vi "Circular Buffer Address.vi"(5 "Reset?":bool, 7 "Starting Address":u32, 11 "Records to Acquire":u32) -> (3 "Address":u32)   [LabVIEW 2012]
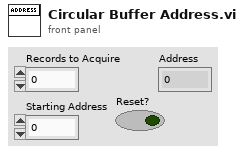
[diagram p1: front panel]
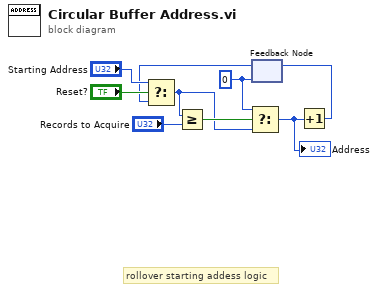
[diagram p0: block diagram]
diagram:
  w9 = u32 0
  # "rollover starting addess logic"
  n1 = feedback #1(w9) -> (w2:u32)
  n2 = Select(t="Starting Address", s="Reset?", f=w2) -> (s? t:f=w1:u32)
  n3 = Greater Or Equal?(x=w1, y="Records to Acquire") -> (x >= y?=w8:bool)
  n4 = Select(t=w9, s=w8, f=w1) -> (s? t:f=w3:u32)
  "Address" <- w3
  n5 = Increment(x=w3) -> (x+1=w6:u32)
  n6 = feedback-in #1(w6) -> ()
